vi "Is Reentrant Measurement.vi"(8 "error in (no error)":errorcluster, 11 "measurement plugin service in":refnum<class "Measurement Plugin Service.lvclass">) -> (0 "error out":errorcluster, 1 "is reentrant":bool, 3 "measurement plugin service out":refnum<class "Measurement Plugin Service.lvclass">)   [LabVIEW 2021, in "NI Measurement Plug-In SDK.lvlib" / "Measurement Plugin Service.lvclass"]
uses:
  Measurement Plugin Service.lvclass
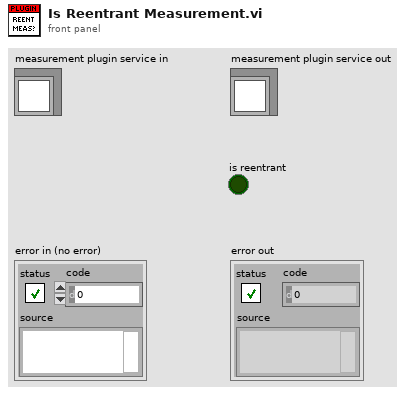
[diagram p1: front panel]
types:
  T1 = typedef "NI Measurement Plug-In SDK.lvlib/Measurement Plugin Service.lvclass/Plugin Paths.ctl" = cluster{"get service descriptor VI path":path, "get type specializations VI path":path, "get UI details VI path":path, "measurement logic VI path":path, "measurement configuration ctl path":path, "measurement results ctl path":path}
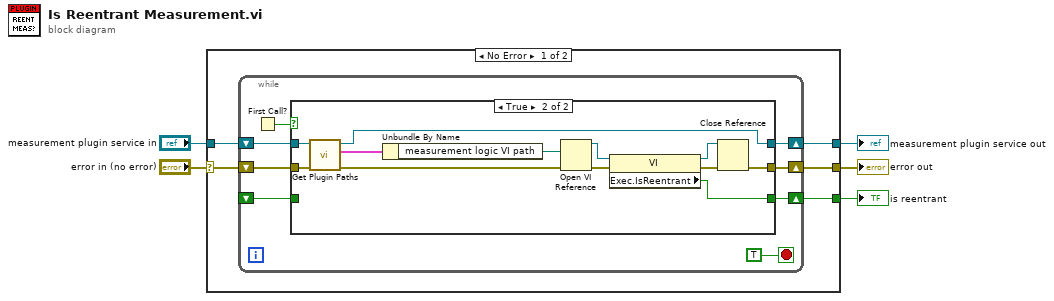
[diagram p0: block diagram]
diagram:
  n1 = case shown="No Error" "error in (no error)" {
    selector: "error in (no error)" -> [w9 w35]
    tunnel: [w7 w35] -> w4
    tunnel: [w8 w34] -> w2
    tunnel: "measurement plugin service in" -> [w10 w34]
    tunnel: [w6 _] -> w1
    frame No Error {
      n2 = while {
        shift-right: [w16] -> w8
        shift-left: w10 -> [w18]
        shift-right: [w15] -> w7
        shift-left: w9 -> [w17]
        shift-right: [w14] -> w6
        shift-left: _ -> [w11]
        stop <- TRUE stop-if-true
        n3 = First Call?() -> (First Call?: T/F=w13:bool)
        n4 = case shown="True" w13 {
          tunnel: w18 -> [w19 w33]
          tunnel: w17 -> [w20 w32]
          tunnel: [w19 w30] -> w16
          tunnel: [w20 w23] -> w15
          tunnel: [w21 w22] -> w14
          tunnel: w11 -> [w21 _]
          frame False {
          }
          frame True {
            n5 = call-dynamic "Get Plugin Paths.vi"("error in"=w32, "measurement plugin service in"=w33) -> ("error out"=w28:errorcluster, "plugin paths"=w31:T1, "measurement plugin service out"=w30:refnum<class "Measurement Plugin Service.lvclass">)  [unwired: 7 in]
            n6 = Unbundle By Name(w31) -> ("measurement logic VI path"=w29:path)
            n7 = Open VI Reference(vi path=w29, error in (no error)=w28) -> (vi reference=w27:refnum<vi>, error out=w26:errorcluster)  [unwired: 4 in]
            n8 = property class="VI"(reference=w27, error in=w26) -> (reference out=w24:refnum<vi>, error out=w25:errorcluster, "Exec.IsReentrant"=w22:bool)
            n9 = Close Reference(reference=w24, error in (no error)=w25) -> (error out=w23:errorcluster)
          }
        }
      }
    }
    frame Error {
    }
  }
  "error out" <- w4
  "measurement plugin service out" <- w2
  "is reentrant" <- w1
